vi "FPGA GPS Test.vi"() -> ()   [LabVIEW 2009]
uses:
  <vilib>/rvi/interface/nirviOpenFPGA/nirviOpenFPGA.xnode
  <vilib>/userDefined/High Color/nirio_resource_hc.ctl
  <vilib>/rvi/interface/nirviReadWriteControl/nirviReadWriteControl.xnode
  <vilib>/rvi/interface/nirviCloseFPGA/nirviCloseFPGA.xnode
  FPGA Bitfiles/Q_IGVC_2010.lvproj_FPGA Target_GPS_2 Port 1 w Com~87.lvbitx
  <vilib>/RVI Host/nirviSupport.llb/nirviErrorClusterFromErrorCode.vi
  <vilib>/rvi/errors/niLvFpgaWhatHappensToTopLevelVI.ctl
  <vilib>/rvi/interface/common/niFpgaNodeNameForErrorReporting.ctl
  <vilib>/rvi/errors/niLvFpgaAdjustHostInterfaceError.vi
  <vilib>/FPGAPlugInAG/cRIO-9113/nirviIntfClose_cRIO-9113.vi
panel:
  out "error out":errorcluster
  out "Current Time":timestamp format="%<%I:%M:%S%2u %p>T"
  out "VI Start Time":timestamp format="%<%I:%M:%S%2u %p>T"
  out "New GPS Data":bool
  out "Bytes at Port?":bool
  in  "stop":bool
  out "Longitude":dbl format="%#_14g"
  out "Latitude":dbl format="%#_14g"
  out "Time":dbl format="%#_14g"
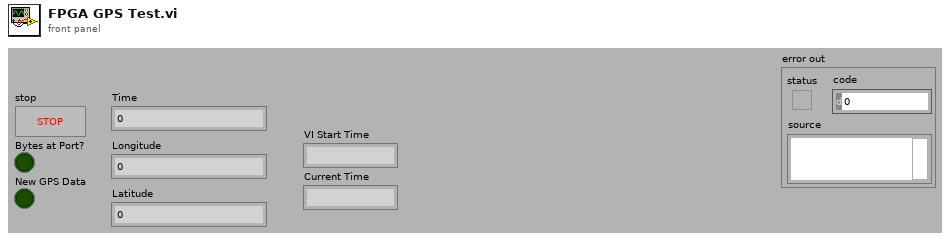
[diagram p1: front panel]
types:
  T1 = typedef "nirio_resource_hc.ctl" = tag
  T2 = typedef "niFpgaNodeNameForErrorReporting.ctl" = enum16{"Open FPGA VI Reference", "Read/Write Control", "Invoke Method: Abort", "Invoke Method: Acknowledge IRQ", "Invoke Method: Download", "Invoke Method: FIFO.Configure", "Invoke Method: FIFO.Read", "Invoke Method: FIFO.Start", "Invoke Method: FIFO.Stop", "Invoke Method: FIFO.Write", "Invoke Method: Reset", "Invoke Method: Run", "Invoke Method: Wait on IRQ", "Close FPGA VI Reference"}
  T3 = typedef "niLvFpgaWhatHappensToTopLevelVI.ctl" = enum16{"top level VI scripted behind XNode", "top level VI inlined behind XNode"}
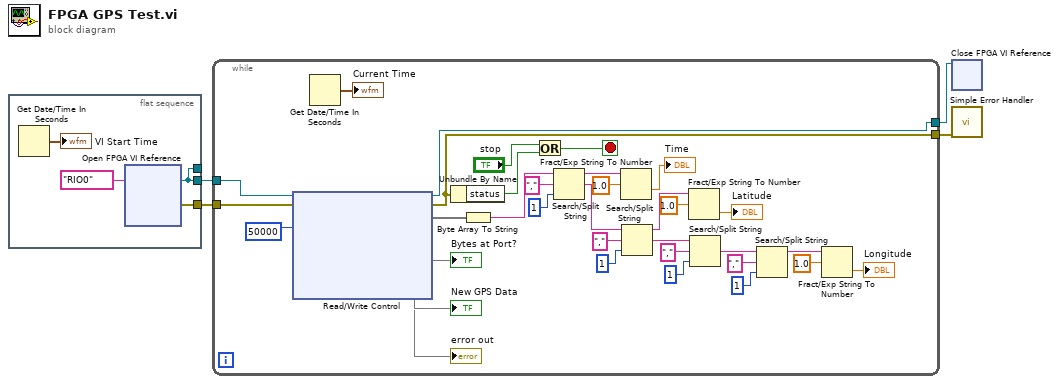
[diagram p0: block diagram]
diagram:
  n1 = flat-sequence {
    tunnel: [w5] -> _
    tunnel: [w7] -> w1
    tunnel: [w5] -> w2
    frame #0 {
      n2 = Get Date/Time In Seconds() -> (seconds since 1Jan1904=→"VI Start Time":timestamp)
      n3 = xnode "Open FPGA VI Reference"("resource name"=T1 "RIO0") -> ("FPGA VI Reference Out"=w5:refnum<k20>, "error out"=w7:errorcluster)  [unwired: 1 in]
    }
  }
  n4 = while {
    tunnel: w2 -> [w43]
    tunnel: w1 -> [w22]
    tunnel: [w15] -> w4
    tunnel: [w11] -> w3
    stop <- w16 stop-if-true
    n5 = xnode "Read/Write Control"("FPGA VI Reference In"=w43, "error in"=w22, "GPS Read Timeout (us)"=50000) -> ("FPGA VI Reference Out"=w11:refnum<k20>, "error out"=w15:errorcluster, "GPS Data"=w23:void[], "Bytes at Port?"=→"Bytes at Port?", "New GPS Data"=→"New GPS Data", "error out"=→"error out")  [unwired: 1 out]
    n6 = Get Date/Time In Seconds() -> (seconds since 1Jan1904=→"Current Time":timestamp)
    n7 = Unbundle By Name(w15) -> ("status"=w14:bool)
    n8 = Byte Array To String(unsigned byte array=w23) -> (string=w12:string)
    n9 = Or(x="stop", y=w14) -> (x .or. y?=w16:bool)
    n10 = Search/Split String(string=w12, search string/char (-)=",", offset (0)=1) -> (substring before match=w29:string, match + rest of string=w36:string)  [unwired: 1 out]
    n11 = Fract/Exp String To Number(string=w29, offset=1.0 ("default (0 I32)")) -> (number=→"Time":dbl)  [unwired: 2 in, 1 out]
    n12 = Search/Split String(string=w36, search string/char (-)=",", offset (0)=1) -> (substring before match=w31:string, match + rest of string=w35:string)  [unwired: 1 out]
    n13 = Fract/Exp String To Number(string=w31, offset=1.0 ("default (0 DBL)")) -> (number=→"Latitude":dbl)  [unwired: 2 in, 1 out]
    n14 = Search/Split String(string=w35, search string/char (-)=",", offset (0)=1) -> (match + rest of string=w32:string)  [unwired: 2 out]
    n15 = Search/Split String(string=w32, search string/char (-)=",", offset (0)=1) -> (substring before match=w21:string)  [unwired: 2 out]
    n16 = Fract/Exp String To Number(string=w21, offset=1.0 ("default (0 I32)")) -> (number=→"Longitude":dbl)  [unwired: 2 in, 1 out]
  }
  n17 = xnode "Close FPGA VI Reference"("FPGA VI Reference In"=w3) -> ()  [unwired: 1 in, 1 out]
  n18 = call <vilib>:"Simple Error Handler.vi"("error in (no error)"=w4) -> ()  [unwired: 4 in, 5 out]
